vi "Example4.vi"() -> ()   [LabVIEW 2021]
doc: "Example of object polymorphism in LabVIEW. Comments in Polish."
uses:
  Astromech droid/Astromech droid.lvclass
  BattleDroid/BattleDroid.lvclass
  MedicalDroid/MedicalDroid.lvclass
  Droid/Droid.lvclass
panel:
  in  "BattleDroid":refnum<class "BattleDroid.lvclass">
  out "Error Out":errorcluster
  in  "AstromechDroid":refnum<class "Astromech droid.lvclass">
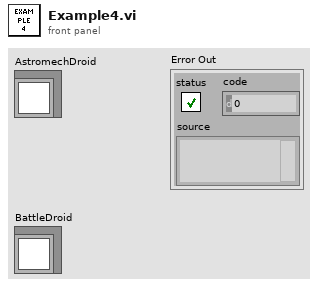
[diagram p1: front panel]
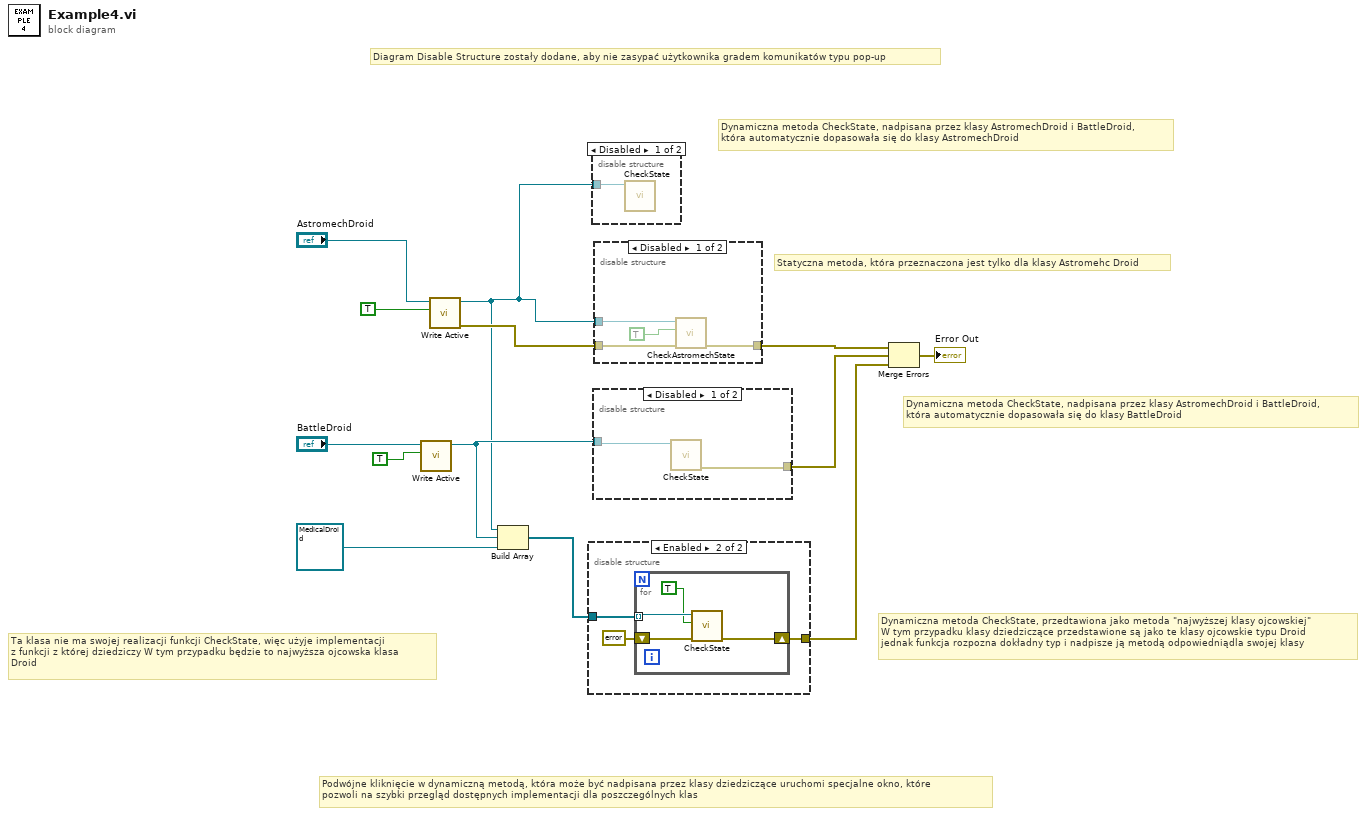
[diagram p0: block diagram]
diagram:
  # "Diagram Disable Structure zostały dodane, aby nie zasypać użytkownika gradem komunikatów typu pop-up"
  # "Ta klasa nie ma swojej realizacji funkcji CheckState, więc użyje implementacji\nz funkcji z której dziedziczy W tym przypadku będzie to najwyższa ojcowska klasa\nDroid"
  # "Podwójne kliknięcie w dynamiczną metodą, która może być nadpisana przez klasy dziedziczące uruchomi specjalne okno, które\npozwoli na szybki przegląd dostępnych implementacji dla poszczególnych klas"
  # "Dynamiczna metoda CheckState, przedtawiona jako metoda \"najwyższej klasy ojcowskiej\" \nW tym przypadku klasy dziedziczące przedstawione są jako te klasy ojcowskie typu Droid \njednak funkcja rozpozna dokładny typ i nadpisze ją metodą odpowiedniądla swojej klasy"
  # "Dynamiczna metoda CheckState, nadpisana przez klasy AstromechDroid i BattleDroid,\nktóra automatycznie dopasowała się do klasy BattleDroid"
  # "Statyczna metoda, która przeznaczona jest tylko dla klasy Astromehc Droid"
  # "Dynamiczna metoda CheckState, nadpisana przez klasy AstromechDroid i BattleDroid,\nktóra automatycznie dopasowała się do klasy AstromechDroid"
  n1 = call-dynamic "Write Active.vi"("Active"=TRUE, "Droid in"="BattleDroid") -> ("Droid out"=w7:refnum<class "BattleDroid.lvclass">)  [unwired: 8 in, 1 out]
  n2 = call-dynamic "Write Active.vi"("Active"=TRUE, "Droid in"="AstromechDroid") -> ("error out"=w12:errorcluster, "Droid out"=w5:refnum<class "Astromech droid.lvclass">)  [unwired: 8 in]
  n3 = Build Array(w5, w7, refnum<class "MedicalDroid.lvclass"> refnum ("MedicalDroid.lvclass")) -> (w9:refnum<class "Droid.lvclass">[])
  n4 = disable-structure shown="Enabled" {
    disable-tunnel: w9 -> [_ w16]
    disable-tunnel: [_ w14] -> w1
    frame Disabled {
    }
    frame Enabled {
      n5 = for {
        tunnel: w16 -> [w20] mode=indexing
        shift-right: [w18] -> w14
        shift-left: errorcluster {"status"=FALSE, "code"=0, "source"=""} ("Error Out") -> [w17]
        n6 = call-dynamic "CheckState.vi"("Error In"=w17, "With sound?"=TRUE, "Droid in"=w20) -> ("Error Out"=w18:errorcluster)  [unwired: 7 in, 1 out]
      }
    }
  }
  n7 = disable-structure shown="Disabled" {
    disable-tunnel: w5 -> [w21 _]
    frame Disabled {
      n8 = call-dynamic "CheckState.vi"("Astromech droid in"=w21) -> ()  [unwired: 9 in, 2 out]
    }
    frame Enabled {
    }
  }
  n9 = disable-structure shown="Disabled" {
    disable-tunnel: w7 -> [w23 _]
    disable-tunnel: [w22 _] -> w2
    frame Disabled {
      n10 = call-dynamic "CheckState.vi"("BattleDroid in"=w23) -> ("Error Out"=w22:errorcluster)  [unwired: 9 in, 1 out]
    }
    frame Enabled {
    }
  }
  n11 = disable-structure shown="Disabled" {
    disable-tunnel: w12 -> [w26 _]
    disable-tunnel: [w25 _] -> w11
    disable-tunnel: w5 -> [w24 _]
    frame Disabled {
      n12 = call "CheckAstromechState.vi"("Error In"=w26, "With sound?"=TRUE, "Astromech droid In"=w24) -> ("Error Out"=w25:errorcluster)  [unwired: 7 in, 1 out]
    }
    frame Enabled {
    }
  }
  n13 = Merge Errors(w11, w2, w1) -> (→"Error Out":errorcluster)
